vi "Render ESP Error Handler.vi"(0 "LabVIEW Web Service Request":refnum<class "Web Request.lvclass">, 1 "Show Error? (T)":bool=TRUE, 5 "Message (empty)":string, 7 "Link":string, 11 "error in (no error)":errorcluster) -> (4 "LabVIEW Web Service Request out":refnum<class "Web Request.lvclass">, 15 "error out":errorcluster)   [LabVIEW 2014]
doc: "This VI is used for all HTTP Method VIs to handle errors during a request. It uses an ESP script to output the error message."
uses:
  <vilib>/wsapi/Web Request.lvclass
  <vilib>/Utility/error.llb/DialogType.ctl
  <vilib>/wsapi/class/subVIs/Set String ESP Variable.vi
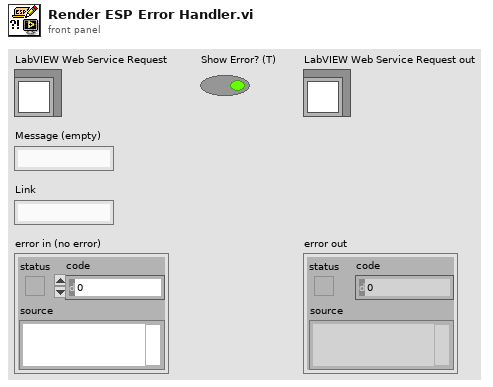
[diagram p1: front panel]
types:
  T1 = typedef "DialogType.ctl" = u16
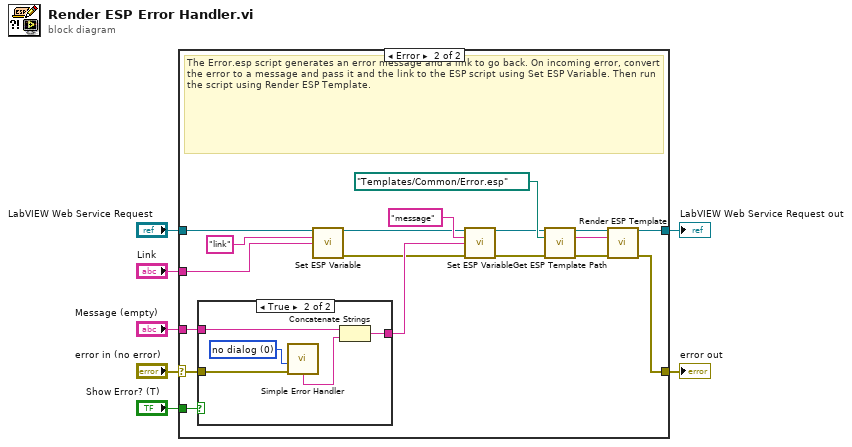
[diagram p0: block diagram]
diagram:
  n1 = case shown="Error" "error in (no error)" {
    selector: "error in (no error)" -> [w9 w24]
    tunnel: [w9 w20] -> w6
    tunnel: "LabVIEW Web Service Request" -> [w8 w15]
    tunnel: [w8 w11] -> w4
    tunnel: "Link" -> [_ w26]
    tunnel: "Message (empty)" -> [_ w23]
    tunnel: "Show Error? (T)" -> [_ w19]
    frame No Error {
      # "Nothing to do if there is not an error."
    }
    frame Error {
      # "The Error.esp script generates an error message and a link to go back. On incoming error, convert the error to a message and pass it and the link to the ESP script using Set ESP Variable. Then run the script using Render ESP Template."
      n2 = case shown="True" w19 {
        tunnel: w24 -> [_ w33]
        tunnel: w23 -> [w28 w32]
        tunnel: [w28 w29] -> w22
        frame False {
        }
        frame True {
          w31 = T1 0 items=["no dialog", "OK message", "continue or stop message", "OK message + warnings", "continue/stop + warnings"] ("type of dialog (OK msg:1)")
          n3 = call <vilib>:"Simple Error Handler.vi"("type of dialog (OK msg:1)"=w31, "error in (no error)"=w33) -> ("message"=w30:string)  [unwired: 3 in, 4 out]
          n4 = Concatenate Strings(w32, w30) -> (w29:string)
        }
      }
      n5 = call-poly <vilib>:"Set ESP Variable.vi"("LabVIEW Web Service Request"=w15, "key"="link", "value"=w26) -> ("LabVIEW Web Service Request out"=w14:refnum<class "Web Request.lvclass">, "error out"=w10:errorcluster)  [unwired: 11 in]
      n6 = call-poly <vilib>:"Set ESP Variable.vi"("LabVIEW Web Service Request"=w14, "key"="message", "value"=w22, "error in (no error)"=w10) -> ("LabVIEW Web Service Request out"=w13:refnum<class "Web Request.lvclass">, "error out"=w21:errorcluster)  [unwired: 10 in]
      n7 = call "Get ESP Template Path.vi"("LabVIEW Web Service Request"=w13, "Relative Template Path"=path "Templates/Common/Error.esp", "error in (no error)"=w21) -> ("LabVIEW Web Service Request out"=w12:refnum<class "Web Request.lvclass">, "Template Name"=w17:string, "error out"=w18:errorcluster)  [unwired: 10 in]
      n8 = call <vilib>:"Render ESP Template.vi"("LabVIEW Web Service Request"=w12, "espName"=w17, "error in (no error)"=w18) -> ("LabVIEW Web Service Request out"=w11:refnum<class "Web Request.lvclass">, "error out"=w20:errorcluster)  [unwired: 11 in]
    }
  }
  "error out" <- w6
  "LabVIEW Web Service Request out" <- w4
